vi "PH_Beckhoff_PP_PU.handle Trigger.vi"(0 "i ref in":refnum<vi>, 4 "Values":T2, 5 "error in":errorcluster, 7 "Values changed at":T1) -> (14 "i ref out":refnum<vi>, 19 "error out":errorcluster)   [LabVIEW 2014, in "PH_Beckhoff_PP_PU.lvlib"]
doc: "This VI handles the incoming information about Trigger inputs: If the value or quality changed, these are set to own attributes and the scaled information is published via DIM."
uses:
  PH_Beckhoff_PP_PU.lvlib
  PH_Beckhoff/PH_Beckhoff.Values.ctl
  PH_Beckhoff/PH_Beckhoff.Sonderklemmen Inputs.ctl
  PH_Beckhoff/PH_Beckhoff.Analog Inputs.ctl
  PH_Beckhoff/PH_Beckhoff.Scaling Type.ctl
  PH_Beckhoff/PH_Beckhoff.Analog Outputs.ctl
  PH_Beckhoff/PH_Beckhoff.Digital Inputs.ctl
  PH_Beckhoff/PH_Beckhoff.Digital Outputs.ctl
  PH_Basics/PH_StatusHandler/PH_StatusHandler.Status.ctl
  PH_Basics/PH_StatusHandler/PH_StatusHandler.lvlib
  CSlibraries-extern/DimLVEvent/LVDimInterface/LVDimInterface.lvlib
  PH_Basics/PH_Common/PH_Common.lvlib
  PH_Beckhoff/PH_Beckhoff.lvlib
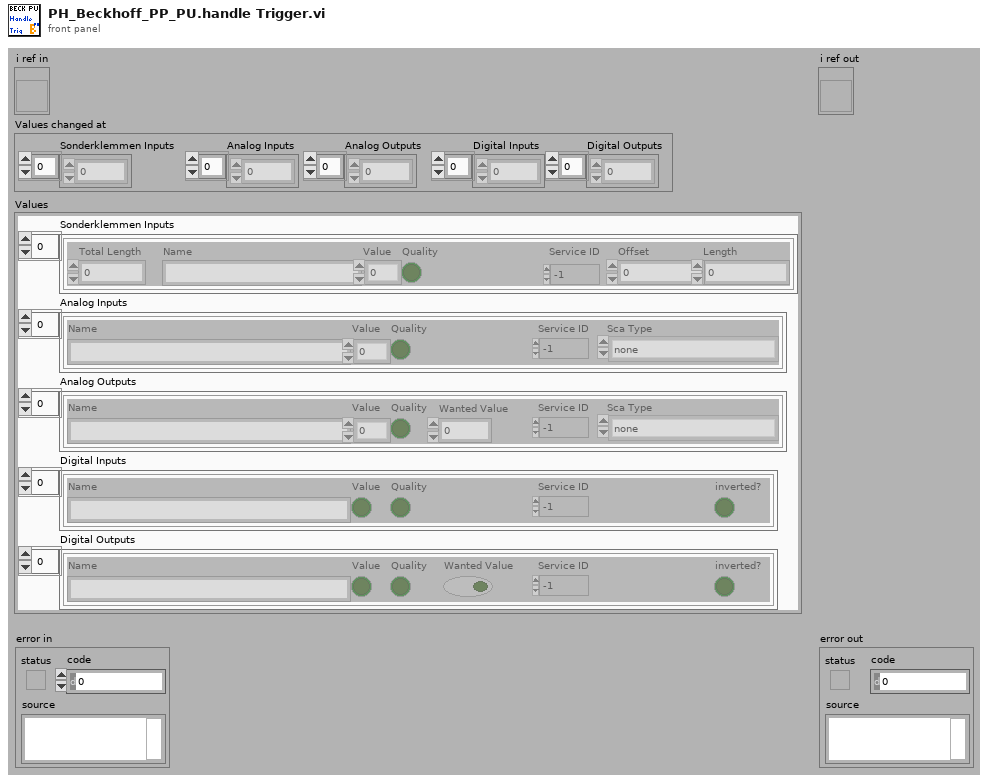
[diagram p1: front panel]
types:
  T1 = cluster{"Sonderklemmen Inputs":i32[], "Analog Inputs":i32[], "Analog Outputs":i32[], "Digital Inputs":i32[], "Digital Outputs":i32[]}
  T2 = typedef "PH_Beckhoff.lvlib/PH_Beckhoff.Values.ctl" = cluster{"Sonderklemmen Inputs":T3, "Analog Inputs":T4, "Analog Outputs":T6, "Digital Inputs":T7, "Digital Outputs":T8}
  T3 = typedef "PH_Beckhoff.lvlib/PH_Beckhoff.Sonderklemmen Inputs.ctl" = cluster{"Total Length":u32, "Name":string, "Value":u64, "Quality":bool, "Service ID":i32, "Offset":u32, "Length":u32}[]
  T4 = typedef "PH_Beckhoff.lvlib/PH_Beckhoff.Analog Inputs.ctl" = cluster{"Name":string, "Value":u32, "Quality":bool, "Service ID":i32, "Sca Type":T5}[]
  T5 = typedef "PH_Beckhoff.lvlib/PH_Beckhoff.Scaling Type.ctl" = enum16{"none", "0 ... 15 Bit -> 0 ... 5", "0 ... 15 Bit -> 0 ... 10", "0 ... 15 Bit -> 0 ... 25", "0 ... 15 Bit -> 4 ... 20", "0 ... 15 Bit -> 0 ... 1", "0 ... 15 Bit -> 0 ... 20000", "0 ... 15 Bit -> 0 ... 24000"}
  T6 = typedef "PH_Beckhoff.lvlib/PH_Beckhoff.Analog Outputs.ctl" = cluster{"Name":string, "Value":u32, "Quality":bool, "Wanted Value":u32, "Service ID":i32, "Sca Type":T5}[]
  T7 = typedef "PH_Beckhoff.lvlib/PH_Beckhoff.Digital Inputs.ctl" = cluster{"Name":string, "Value":bool, "Quality":bool, "Service ID":i32, "inverted?":bool}[]
  T8 = typedef "PH_Beckhoff.lvlib/PH_Beckhoff.Digital Outputs.ctl" = cluster{"Name":string, "Value":bool, "Quality":bool, "Wanted Value":bool, "Service ID":i32, "inverted?":bool}[]
  T9 = typedef "PH_Beckhoff_PP_PU.lvlib/PH_Beckhoff_PP_PU.i attribute.ctl" = cluster{"HV Meas":cluster{"Input GUI Ref":refnum<vi>, "Voltage Service ID":i32, "Voltage [V]":dbl, "Quality":bool, "# in Data":i32}[], "Trigger":cluster{"Status":cluster{"GUI Ref":refnum<vi>, "Status Service ID":i32, "Status":T10}, "last shot:":cluster{"GUI Ref":refnum<vi>, "Service ID":i32, "Time":string}, "DIs":cluster{"triggered":cluster{"GUI Ref":refnum<vi>, "# in Data":i32}, "fired":cluster{"GUI Ref":refnum<vi>, "# in Data":i32}}, "GUI Ref Indicator":refnum<vi>}[], "RR":cluster{"Status":cluster{"GUI Ref":refnum<vi>, "Status Service ID":i32, "Status":T10}, "DIs":cluster{"closed":cluster{"GUI Ref":refnum<vi>, "# in Data":i32}, "open":cluster{"GUI Ref":refnum<vi>, "# in Data":i32}}, "Close":cluster{"GUI Ref":refnum<vi>, "# in Data":i32}, "GUI Ref Indicator":refnum<vi>}[], "Igni":cluster{"Status":cluster{"GUI Ref":refnum<vi>, "Status Service ID":i32, "Status":T10}, "DIs":cluster{"heating on":cluster{"GUI Ref":refnum<vi>, "# in Data":i32}, "water on":cluster{"GUI Ref":refnum<vi>, "# in Data":i32}}, "Device on":cluster{"GUI Ref":refnum<vi>, "# in Data":i32}, "GUI Ref Indicator":refnum<vi>}[], "PSU":cluster{"Status":cluster{"GUI Ref":refnum<vi>, "Status Service ID":i32, "Status":T10}, "Limit Service ID":i32, "DIs":cluster{"inhibit":cluster{"GUI Ref":refnum<vi>, "# in Data":i32}, "end of charge":cluster{"GUI Ref":refnum<vi>, "# in Data":i32}, "HV on":cluster{"GUI Ref":refnum<vi>, "# in Data":i32}, "overtemp":cluster{"GUI Ref":refnum<vi>, "# in Data":i32}, "interlock":cluster{"GUI Ref":refnum<vi>, "# in Data":i32}, "load fault":cluster{"GUI Ref":refnum<vi>, "# in Data":i32}, "sum fault":cluster{"GUI Ref":refnum<vi>, "# in Data":i32}, "HV off":cluster{"GUI Ref":refnum<vi>, "# in Data":i32}, "DC ok":cluster{"GUI Ref":refnum<vi>, "# in Data":i32}}, "AIs":cluster{"voltage":cluster{"GUI Ref":refnum<vi>, "# in Data":i32}, "current":cluster{"GUI Ref":refnum<vi>, "# in Data":i32}}, "DAs":cluster{"inhibit":cluster{"GUI Ref":refnum<vi>, "# in Data":i32}, "interlock":cluster{"GUI Ref":refnum<vi>, "# in Data":i32}, "HV on":cluster{"GUI Ref":refnum<vi>, "# in Data":i32}, "Reset":cluster{"GUI Ref":refnum<vi>, "# in Data":i32}}, "AAs":cluster{"Voltage to set":cluster{"GUI Ref":refnum<vi>, "# in Data":i32}}, "GUI Ref Indicator":refnum<vi>}[], "reconfigured":cluster{"?":bool, "GUI Ref":refnum<vi>}, "PU Rack Type":T11, "HV Meas Info":T12, "PSU Info":T13}
  T10 = typedef "PH_StatusHandler.lvlib/PH_StatusHandler.Status.ctl" = i16
  T11 = typedef "PH_Beckhoff_PP_PU.lvlib/PH_Beckhoff_PP_PU.PU Rack Type.ctl" = enum16{"no Info", "PA 19mm", "PA 45mm", "MA PU 1 and 2", "MA PU 3 and 4", "MA PU 5 and 6", "MA FR and PILC"}
  T12 = typedef "PH_Beckhoff_PP_PU.lvlib/PH_Beckhoff_PP_PU.HV Meas Info.ctl" = cluster{"Period Time [s]":dbl, "Subtractor 1 [Hz]":dbl, "Devider 1 [Hz/kV]":dbl, "Subtractor 2 [Hz]":dbl, "Devider 2 [Hz/kV]":dbl}
  T13 = typedef "PH_Beckhoff_PP_PU.lvlib/PH_Beckhoff_PP_PU.PSU Info.ctl" = cluster{"Limits 1 [V]":cluster{"Lower":dbl, "Upper":dbl}, "Limits 2 [V]":cluster{"Lower":dbl, "Upper":dbl}}
  T14 = cluster{"Status":cluster{"GUI Ref":refnum<vi>, "Status Service ID":i32, "Status":T10}, "last shot:":cluster{"GUI Ref":refnum<vi>, "Service ID":i32, "Time":string}, "DIs":cluster{"triggered":cluster{"GUI Ref":refnum<vi>, "# in Data":i32}, "fired":cluster{"GUI Ref":refnum<vi>, "# in Data":i32}}, "GUI Ref Indicator":refnum<vi>}[]
  T15 = cluster{"Status":cluster{"GUI Ref":refnum<vi>, "Status Service ID":i32, "Status":T10}, "last shot:":cluster{"GUI Ref":refnum<vi>, "Service ID":i32, "Time":string}, "DIs":cluster{"triggered":cluster{"GUI Ref":refnum<vi>, "# in Data":i32}, "fired":cluster{"GUI Ref":refnum<vi>, "# in Data":i32}}, "GUI Ref Indicator":refnum<vi>}
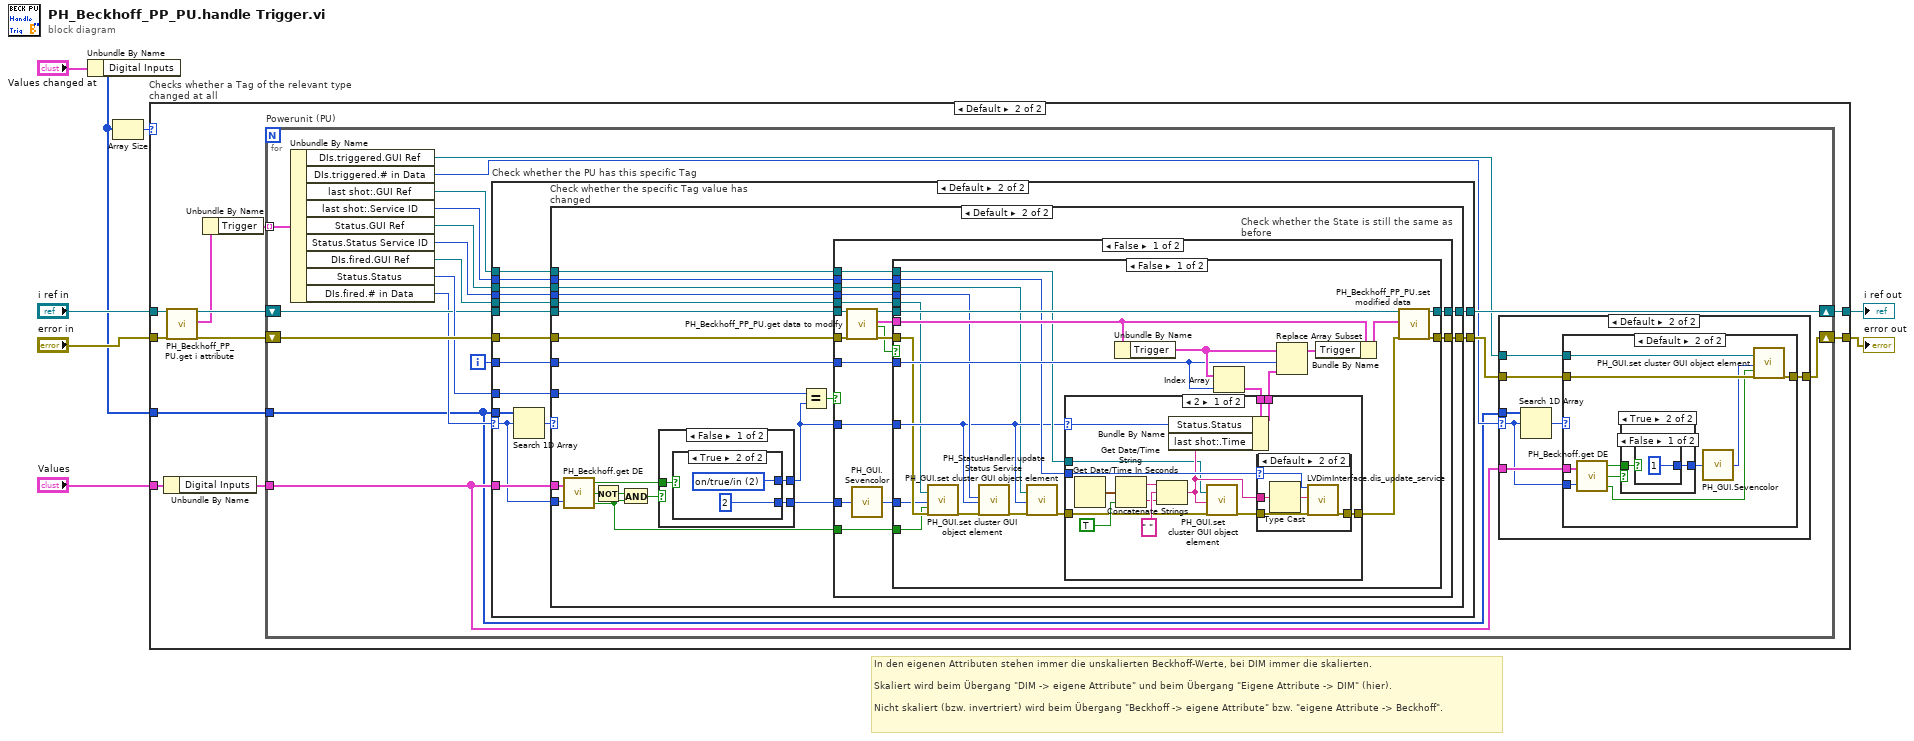
[diagram p0: block diagram]
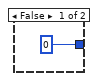
[diagram p5: hidden frame]
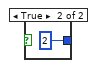
[diagram p6: hidden frame]
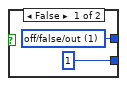
[diagram p9: hidden frame]
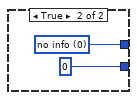
[diagram p10: hidden frame]
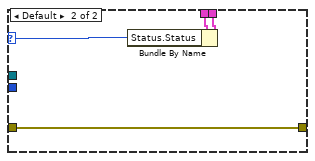
[diagram p12: hidden frame]
diagram:
  # "In den eigenen Attributen stehen immer die unskalierten Beckhoff-Werte, bei DIM immer die skalierten.\n\nSkaliert wird beim Übergang \"DIM -> eigene Attribute\" und beim Übergang \"Eigene Attribute -> DIM\" (hier).\n\nNicht skaliert (bzw. invertriert) wird beim Übergang \"Beckhoff -> eigene Attribute\" bzw. \"eigene Attribute -> Beckhoff\"."
  n1 = Unbundle By Name("Values changed at") -> ("Digital Inputs"=w1:i32[])
  n2 = Array Size(array=w1) -> (size(s)=w2:i32)
  n3 = case "Checks whether a Tag of the relevant type changed at all" shown="Default" w2 {
    tunnel: [w10 w21] -> w8
    tunnel: "i ref in" -> [w10 w16]
    tunnel: "error in" -> [w9 w19]
    tunnel: [w9 w12] -> w5
    tunnel: "Values" -> [_ w18]
    tunnel: w1 -> [_ w11]
    frame 0 {
    }
    frame Default {
      n4 = Unbundle By Name(w18) -> ("Digital Inputs"=w20:T7)
      n5 = call "PH_Beckhoff_PP_PU.get i attribute.vi"("i ref in"=w16, "error in (no error)"=w19) -> ("i ref out"=w15:refnum<vi>, "i attribute"=w14:T9, "error out"=w17:errorcluster)  [unwired: 15 in]
      n6 = Unbundle By Name(w14) -> ("Trigger"=w13:T14)
      n7 = for "Powerunit (PU)" {
        shift-right: [w26] -> w12
        shift-left: w17 -> [w37]
        tunnel: w13 -> [w39] mode=indexing
        shift-right: [w34] -> w21
        shift-left: w15 -> [w35]
        tunnel: w20 -> [w23]
        tunnel: w11 -> [w22]
        i -> [w33]
        n8 = Unbundle By Name(w39) -> ("DIs.triggered.GUI Ref"=w24:refnum<vi>, "DIs.triggered.# in Data"=w25:i32, "last shot:.GUI Ref"=w30:refnum<vi>, "last shot:.Service ID"=w32:i32, "Status.GUI Ref"=w29:refnum<vi>, "Status.Status Service ID"=w38:i32, "DIs.fired.GUI Ref"=w28:refnum<vi>, "Status.Status"=w36:T10, "DIs.fired.# in Data"=w31:i32)
        n9 = case "Check whether the PU has this specific Tag" shown="Default" w31 {
          selector: w31 -> [_ w72]
          tunnel: [w65 w80] -> w27
          tunnel: w38 -> [_ w66]
          tunnel: w37 -> [w65 w79]
          tunnel: w36 -> [_ w78]
          tunnel: w35 -> [w64 w77]
          tunnel: [w64 w76] -> w34
          tunnel: w33 -> [_ w73]
          tunnel: w23 -> [_ w75]
          tunnel: w32 -> [_ w74]
          tunnel: w22 -> [_ w71]
          tunnel: w30 -> [_ w69]
          tunnel: w29 -> [_ w68]
          tunnel: w28 -> [_ w67]
          frame -1 {
          }
          frame Default {
            n10 = Search 1D Array(1D array=w71, element=w72) -> (index of element=w70:i32)  [unwired: 1 in]
            n11 = case "Check whether the specific Tag value has changed" shown="Default" w70 {
              tunnel: [w81 w103] -> w80
              tunnel: w66 -> [_ w102]
              tunnel: w79 -> [w81 w101]
              tunnel: w78 -> [_ w100]
              tunnel: w77 -> [w82 w99]
              tunnel: [w82 w98] -> w76
              tunnel: w75 -> [_ w97]
              tunnel: w74 -> [_ w93]
              tunnel: w73 -> [_ w88]
              tunnel: w72 -> [_ w87]
              tunnel: w69 -> [_ w86]
              tunnel: w68 -> [_ w85]
              tunnel: w67 -> [_ w84]
              frame -1 {
              }
              frame Default {
                n12 = call "PH_Beckhoff.get DE.vi"("Digital Values"=w97, "index of element"=w87) -> ("Value"=w89:bool, "Quality"=w90:bool, "Tag not found"=w83:bool)
                n13 = Not(x=w90) -> (.not. x?=w96:bool)
                n14 = And(x=w96, y=w83) -> (x .and. y?=w94:bool)
                n15 = case shown="False" w94 {
                  tunnel: w89 -> [w106 _]
                  tunnel: [w105 w112] -> w92
                  tunnel: [w104 0 ("State")] -> w91
                  frame False {
                    n16 = case shown="True" w106 {
                      tunnel: [w108 w110] -> w105
                      tunnel: [1 ("State") 2 ("State")] -> w104
                      frame False {
                        w108 = T10 1 items=["no info", "off/false/out", "on/true/in", "Failure", "Alarm", "Status 1", "Status 2", "Status 3"] ("Status")
                      }
                      frame True {
                        w110 = T10 2 items=["no info", "off/false/out", "on/true/in", "Failure", "Alarm", "Status 1", "Status 2", "Status 3"] ("Status")
                      }
                    }
                  }
                  frame True {
                    w112 = T10 0 items=["no info", "off/false/out", "on/true/in", "Failure", "Alarm", "Status 1", "Status 2", "Status 3"] ("Status")
                  }
                }
                n17 = Equal?(x=w100, y=w92) -> (x = y?=w95:bool)
                n18 = case "Check whether the State is still the same as before" shown="False" w95 {
                  tunnel: w93 -> [w130 _]
                  tunnel: [w124 w180] -> w103
                  tunnel: w102 -> [w129 _]
                  tunnel: w101 -> [w128 w180]
                  tunnel: w92 -> [w127 _]
                  tunnel: w99 -> [w125 w181]
                  tunnel: [w122 w181] -> w98
                  tunnel: w88 -> [w120 _]
                  tunnel: w91 -> [w115 _]
                  tunnel: w86 -> [w118 _]
                  tunnel: w85 -> [w117 _]
                  tunnel: w84 -> [w114 _]
                  tunnel: w83 -> [w113 _]
                  frame False {
                    n19 = call "PH_Beckhoff_PP_PU.get data to modify.vi"("i ref in"=w125, "error in (no error)"=w128) -> ("i ref out"=w123:refnum<vi>, "i attribute"=w121:T9, "timed out"=w119:bool, "error out"=w126:errorcluster)  [unwired: 14 in]
                    n20 = call "PH_GUI.Sevencolor.vi"("State"=w115) -> ("Color Box"=w116:u32)
                    n21 = case shown="False" w119 {
                      tunnel: w130 -> [w141 _]
                      tunnel: w129 -> [w145 _]
                      tunnel: w127 -> [w137 _]
                      tunnel: w126 -> [w135 w178]
                      tunnel: [w153 w178] -> w124
                      tunnel: w123 -> [w152 w179]
                      tunnel: [w151 w179] -> w122
                      tunnel: w121 -> [w150 _]
                      tunnel: w120 -> [w146 _]
                      tunnel: w116 -> [w133 _]
                      tunnel: w118 -> [w140 _]
                      tunnel: w117 -> [w136 _]
                      tunnel: w114 -> [w132 _]
                      tunnel: w113 -> [w131 _]
                      frame False {
                        n22 = call "PH_GUI.set cluster GUI object element.vi"("Ctl Refnum"=w132, "Value"=w133, "Blinking? (false)"=w131, "error in"=w135) -> ("error out"=w134:errorcluster)  [unwired: 15 in]
                        n23 = call "PH_StatusHandler.update Status Service.vi"("Service ID"=w145, "Status"=w137, "error in (no error)"=w134) -> ("error out"=w139:errorcluster)  [unwired: 16 in]
                        n24 = call "PH_GUI.set cluster GUI object element.vi"("Ctl Refnum"=w136, "Value"=w137, "error in"=w139) -> ("error out"=w138:errorcluster)  [unwired: 16 in]
                        n25 = Unbundle By Name(w150) -> ("Trigger"=w147:T14)
                        n26 = Index Array(array=w147, index=w146) -> (element=w144:T15)
                        n27 = case shown="2" w137 {
                          selector: w137 -> [w160 w175]
                          tunnel: w138 -> [w157 w174]
                          tunnel: [w158 w174] -> w142
                          tunnel: w144 -> [w162 w177]
                          tunnel: [w161 w176] -> w143
                          tunnel: w141 -> [w159 _]
                          tunnel: w140 -> [w154 _]
                          frame 2 {
                            n28 = Get Date/Time In Seconds() -> (seconds since 1Jan1904=w166:timestamp)
                            n29 = Get Date/Time String(seconds (now)=w166, want seconds? (F)=TRUE) -> (date string=w165:string, time string=w164:string)  [unwired: 1 in]
                            n30 = Concatenate Strings(w165, " " ("string"), w164) -> (w155:string)
                            n31 = Bundle By Name(cluster=w162, "Status.Status"=w160, "last shot:.Time"=w155) -> (w161:T15)
                            n32 = call "PH_GUI.set cluster GUI object element.vi"("Ctl Refnum"=w154, "Value"=w155, "error in"=w157) -> ("error out"=w156:errorcluster)  [unwired: 16 in]
                            n33 = case shown="Default" w159 {
                              selector: w159 -> [_ w171]
                              tunnel: [w168 w172] -> w158
                              tunnel: w156 -> [w168 w173]
                              tunnel: w155 -> [_ w169]
                              frame -1 {
                              }
                              frame Default {
                                n34 = Type Cast(x=w169) -> (*(type *) &x=w170:string)  [unwired: 1 in]
                                n35 = call "LVDimInterface.dis_update_service.vi"("my_serviceID"=w171, "data"=w170, "error in (no error)"=w173) -> ("error out"=w172:errorcluster)  [unwired: 14 in, 2 out]
                              }
                            }
                          }
                          frame Default {
                            n36 = Bundle By Name(cluster=w177, "Status.Status"=w175) -> (w176:T15)
                          }
                        }
                        n37 = Replace Array Subset(array=w147, new element=w143, index=w146) -> (w148:T14)
                        n38 = Bundle By Name(cluster=w150, "Trigger"=w148) -> (w149:T9)
                        n39 = call "PH_Beckhoff_PP_PU.set modified data.vi"("i ref in"=w152, "i attribute"=w149, "error in (no error)"=w142) -> ("i ref out"=w151:refnum<vi>, "error out"=w153:errorcluster)  [unwired: 15 in]
                      }
                      frame True {
                      }
                    }
                  }
                  frame True {
                  }
                }
              }
            }
          }
        }
        n40 = case shown="Default" w25 {
          selector: w25 -> [_ w44]
          tunnel: [w40 w47] -> w26
          tunnel: w27 -> [w40 w46]
          tunnel: w23 -> [_ w45]
          tunnel: w22 -> [_ w43]
          tunnel: w24 -> [_ w41]
          frame -1 {
          }
          frame Default {
            n41 = Search 1D Array(1D array=w43, element=w44) -> (index of element=w42:i32)  [unwired: 1 in]
            n42 = case shown="Default" w42 {
              tunnel: [w48 w51] -> w47
              tunnel: w46 -> [w48 w58]
              tunnel: w45 -> [_ w57]
              tunnel: w44 -> [_ w54]
              tunnel: w41 -> [_ w53]
              frame -1 {
              }
              frame Default {
                n43 = call "PH_Beckhoff.get DE.vi"("Digital Values"=w57, "index of element"=w54) -> ("Value"=w55:bool, "Quality"=w50:bool, "Tag not found"=w49:bool)
                n44 = case shown="True" w50 {
                  tunnel: w55 -> [_ w61]
                  tunnel: [0 ("State") w60] -> w56
                  frame False {
                  }
                  frame True {
                    n45 = case shown="False" w61 {
                      tunnel: [1 ("State") 2 ("State")] -> w60
                      frame False {
                      }
                      frame True {
                      }
                    }
                  }
                }
                n46 = call "PH_GUI.Sevencolor.vi"("State"=w56) -> ("Color Box"=w52:u32)
                n47 = call "PH_GUI.set cluster GUI object element.vi"("Ctl Refnum"=w53, "Value"=w52, "Blinking? (false)"=w49, "error in"=w58) -> ("error out"=w51:errorcluster)  [unwired: 15 in]
              }
            }
          }
        }
      }
    }
  }
  "i ref out" <- w8
  "error out" <- w5
